vi "Dequeue.vi"(8 "error in (no error)":errorcluster, 9 "timeout in ms (-1)":i32=-1, 11 "Message Queue in":refnum<class "Message Queue.lvclass">) -> (0 "error out":errorcluster, 1 "timed out?":bool, 2 "Message out":refnum<class "Abstract Message.lvclass">, 3 "Message Queue out":refnum<class "Message Queue.lvclass">)   [LabVIEW 2027, in "Messaging.lvlib" / "Message Queue.lvclass"]
uses:
  Message Queue.lvclass
  Message/Abstract Message/Abstract Message.lvclass
  Message Queue.lvclass/Message Queue.ctl
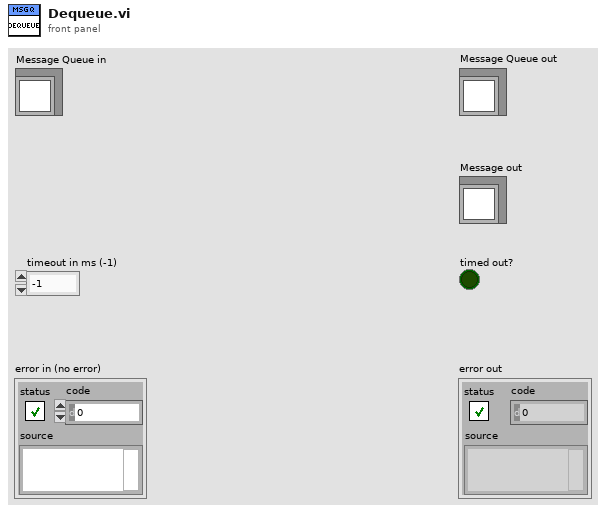
[diagram p1: front panel]
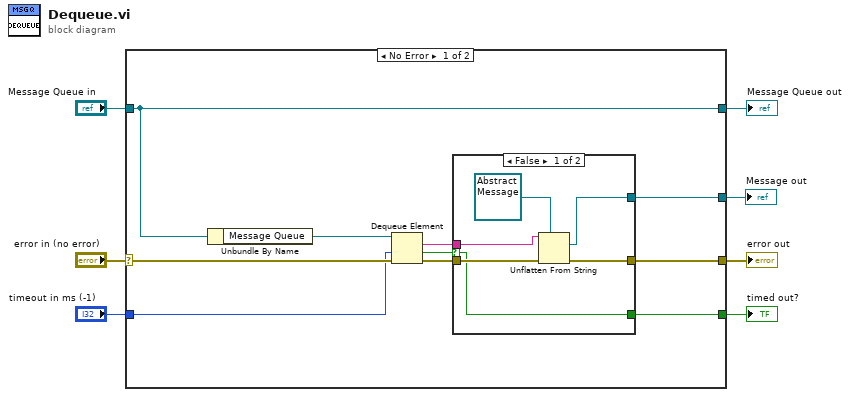
[diagram p0: block diagram]
diagram:
  n1 = case shown="No Error" "error in (no error)" {
    selector: "error in (no error)" -> [w15 w27]
    tunnel: [w13 w27] -> w6
    tunnel: [w17 w26] -> w4
    tunnel: "Message Queue in" -> [w17 w26]
    tunnel: [w11 _] -> w3
    tunnel: "timeout in ms (-1)" -> [w10 _]
    tunnel: [w8 _] -> w1
    frame No Error {
      n2 = Unbundle By Name(w17) -> ("Message Queue"=w16:refnum<queue>)
      n3 = Dequeue Element(queue=w16, timeout in ms (-1)=w10, error in (no error)=w15) -> (element=w12:string, timed out?=w9:bool, error out=w14:errorcluster)  [unwired: 1 out]
      n4 = case shown="False" w9 {
        selector: w9 -> [w18 w24]
        tunnel: w14 -> [w23 w25]
        tunnel: [w22 w25] -> w13
        tunnel: w12 -> [w21 _]
        tunnel: [w19 _] -> w11
        tunnel: [w18 w24] -> w8
        frame False {
          n5 = Unflatten From String(type=refnum<class "Abstract Message.lvclass"> refnum ("Message out"), binary string=w21, error in (no error)=w23) -> (value=w19:refnum<class "Abstract Message.lvclass">, error out=w22:errorcluster)  [unwired: 2 in, 1 out]
        }
        frame True {
        }
      }
    }
    frame Error {
    }
  }
  "error out" <- w6
  "Message Queue out" <- w4
  "Message out" <- w3
  "timed out?" <- w1
